vi "DT3120_Test.vi"() -> ()   [LabVIEW 8.6]
panel:
  out "Image":T1(plugin-control)
  in  "stop":bool
  out "Intensity Graph":u8[][](graph)
  out "Frame Size":T2
  out "CurDevCaps":T3
  out "Active Source":u16
  out "Source List":u16[](array[numeric])
  out "Frame Info":T4
  out "Device List":T5(array[cluster])
  out "Alias List":string[](array[string])
  out "error out":errorcluster
  in  "error in (no error)":errorcluster
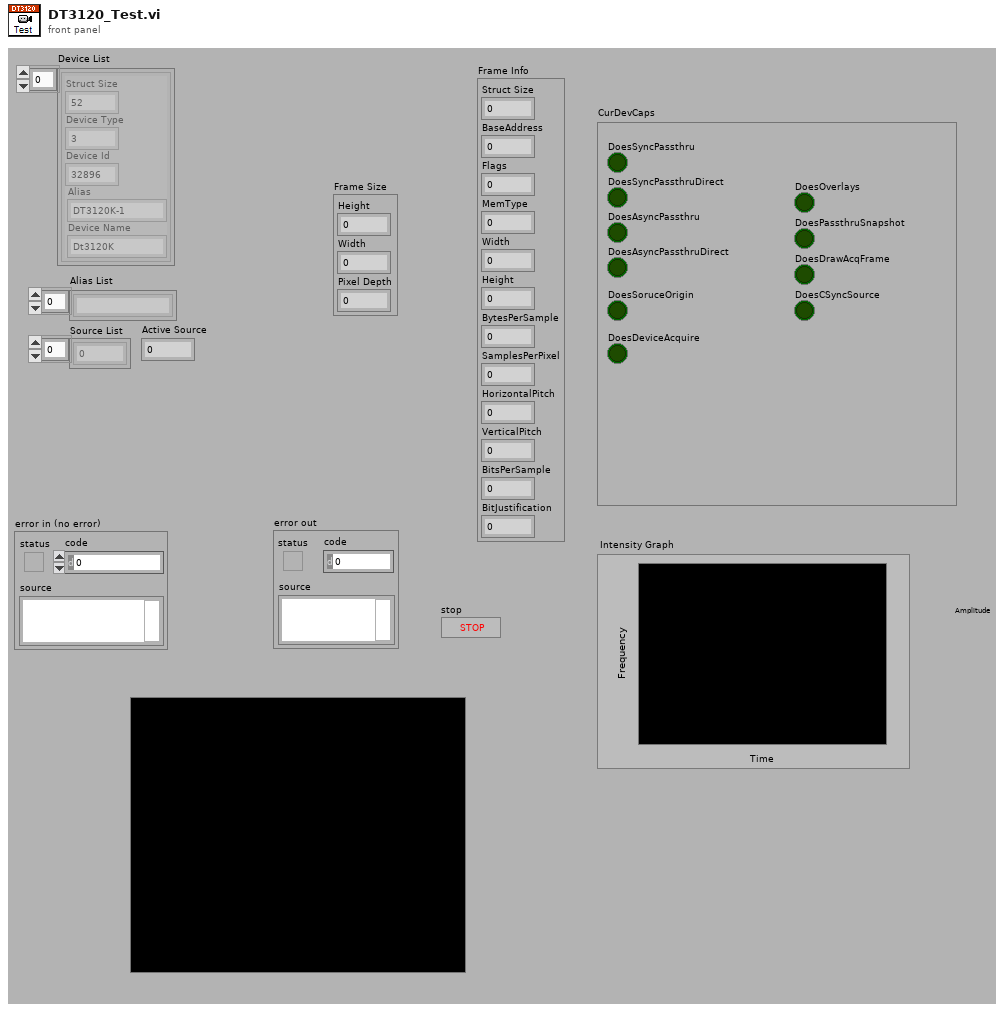
[diagram p1: front panel]
types:
  T1 = typedef "IMAQ Image.ctl" = refnum<image>
  T2 = cluster{"Height":u32, "Width":u32, "Pixel Depth":u32}
  T3 = cluster{"DoesSyncPassthru":bool, "DoesSyncPassthruDirect":bool, "DoesAsyncPassthru":bool, "DoesAsyncPassthruDirect":bool, "DoesSoruceOrigin":bool, "DoesDeviceAcquire":bool, "DoesOverlays":bool, "DoesPassthruSnapshot":bool, "DoesDrawAcqFrame":bool, "DoesCSyncSource":bool}
  T4 = cluster{"Struct Size":u32, "BaseAddress":u32, "Flags":u32, "MemType":u32, "Width":u16, "Height":u16, "BytesPerSample":u16, "SamplesPerPixel":u16, "HorizontalPitch":u16, "VerticalPitch":u16, "BitsPerSample":u16, "BitJustification":u32}
  T5 = cluster{"Struct Size":u32, "Device Type":u32, "Device Id":u32, "Alias":string, "Device Name":string}[]
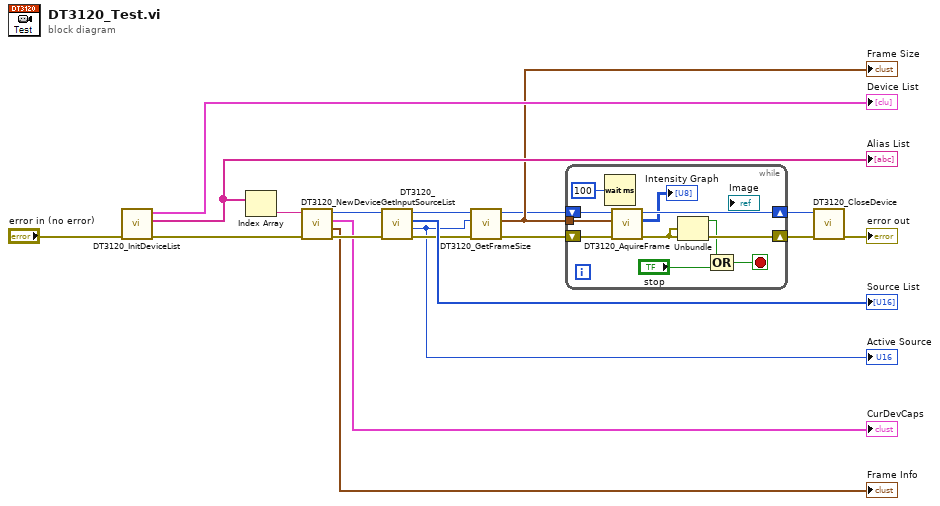
[diagram p0: block diagram]
diagram:
  n1 = call "DT3120_InitDeviceList.vi"("error in (no error)"="error in (no error)") -> ("error out"=w16:errorcluster, "Alias List"=w17:string[], "Device List"=→"Device List":T5)  [unwired: 8 out]
  "Alias List" <- w17
  n2 = Index Array(array=w17) -> (element=w15:string)  [unwired: 1 in]
  n3 = call "DT3120_NewDevice.vi"("error in (no error)"=w16, "Alias"=w15) -> ("error out"=w14:errorcluster, "Frame Info"=→"Frame Info":T4, "CurDevCaps"=→"CurDevCaps":T3, "DevId"=w13:i32)  [unwired: 6 out]
  n4 = call "DT3120_GetInputSourceList.vi"("error in (no error)"=w14, "DevId"=w13) -> ("error out"=w8:errorcluster, "Active Source"=w7:u16, "Source List"=→"Source List":u16[], "DevId (dup)"=w6:i32)  [unwired: 6 out]
  "Active Source" <- w7
  n5 = call "DT3120_GetFrameSize.vi"("error in (no error)"=w8, "Source"=w7, "DevId"=w6) -> ("error out"=w5:errorcluster, "Frame Size"=w3:T2, "DevId (dup)"=w2:i32)  [unwired: 6 in]
  "Frame Size" <- w3
  n6 = while {
    tunnel: w3 -> [w28]
    shift-right: [w23] -> w4
    shift-left: w5 -> [w29]
    shift-right: [w26] -> w1
    shift-left: w2 -> [w27]
    stop <- w20 stop-if-true
    n7 = Wait (ms)(milliseconds to wait=u32 100) -> ()  [unwired: 1 out]
    n8 = call "DT3120_AquireFrame.vi"("error in (no error)"=w29, "Frame Size"=w28, "DevId"=w27) -> ("error out"=w23:errorcluster, "Frame"=→"Intensity Graph":u8[][], "DevId (dup)"=w26:i32)  [unwired: 5 in, 1 out]
    n9 = Unbundle(w23) -> ("status"=w22:bool)  [unwired: 2 out]
    n10 = Compound Arithmetic op=OR(w22, "stop") -> (w20:bool)
  }
  n11 = call "DT3120_CloseDevice.vi"("error in (no error)"=w4, "lpDevId"=w1) -> ("error out"=→"error out":errorcluster)  [unwired: 9 out]
